vi "daqio_Create_Default_Dashboard.vi"(8 "error in":errorcluster, 11 "daq.io type in":T1={"daq.io ref"=refnum, "daq.io API Base"="http://dashboard.daq.io/api/v1", "Device Key"="", "Account ID"="", "online"=TRUE, "SSL"=TRUE, "buffer"=TRUE}) -> (0 "error out":errorcluster, 2 "Dashboard URL":string, 3 "daq.io type out":T1={"daq.io ref"=refnum, "daq.io API Base"="http://dashboard.daq.io/api/v1", "Device Key"="", "Account ID"="", "online"=TRUE, "SSL"=TRUE, "buffer"=TRUE})   [LabVIEW 2013, in "daqio minimal.lvlib"]
doc: "This VI creates a new default dashboard for a specific account and makes it the new default dashboard for the current device."
uses:
  daqio minimal.lvlib
  _typedefs/daqio-Type.ctl
  <vilib>/httpClient/ClientHandle.ctl
  _typedefs/daqio-Device-Just-Dashboards.ctl
  _typedefs/daqio-Device-Dashboards.ctl
  _typedefs/daqio-Device-Put-Dashboards.ctl
  <vilib>/Easy HTTP Client/Easy HTTP.lvlib
  <vilib>/httpClient/LabVIEWHTTPClient.lvlib
panel:
  out "JSON string":string
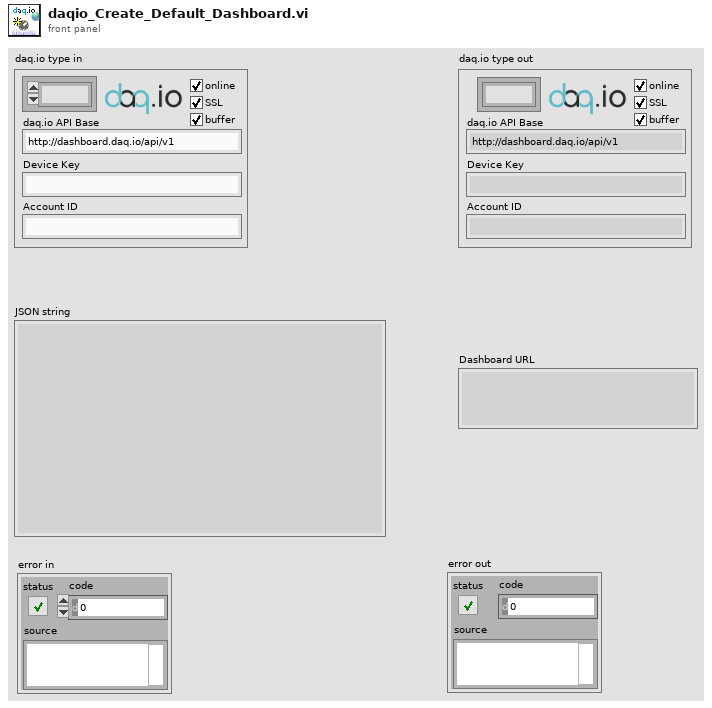
[diagram p1: front panel]
types:
  T1 = typedef "daqio minimal.lvlib/daqio-Type.ctl" = cluster{"daq.io ref":T2, "daq.io API Base":string, "Device Key":string, "Account ID":string, "online":bool, "SSL":bool, "buffer":bool}
  T2 = typedef "LabVIEWHTTPClient.lvlib/ClientHandle.ctl" = refnum<k1>
  T3 = typedef "daqio minimal.lvlib/daqio-Device-Just-Dashboards.ctl" = T4[]
  T4 = typedef "daqio minimal.lvlib/daqio-Device-Dashboards.ctl" = cluster{"active":bool, "definition":string, "_id":string, "label":string}
  T5 = typedef "daqio minimal.lvlib/daqio-Device-Put-Dashboards.ctl" = cluster{"dashboards":T4[]}
  T6 = cluster{"active":bool, "definition":string, "label":string}
  T7 = typedef "daqio minimal.lvlib/daqio-Device-Channels.ctl" = T8[]
  T8 = typedef "daqio minimal.lvlib/daqio-Channels.ctl" = cluster{"key":string, "label":string, "data_type":string, "id":string}
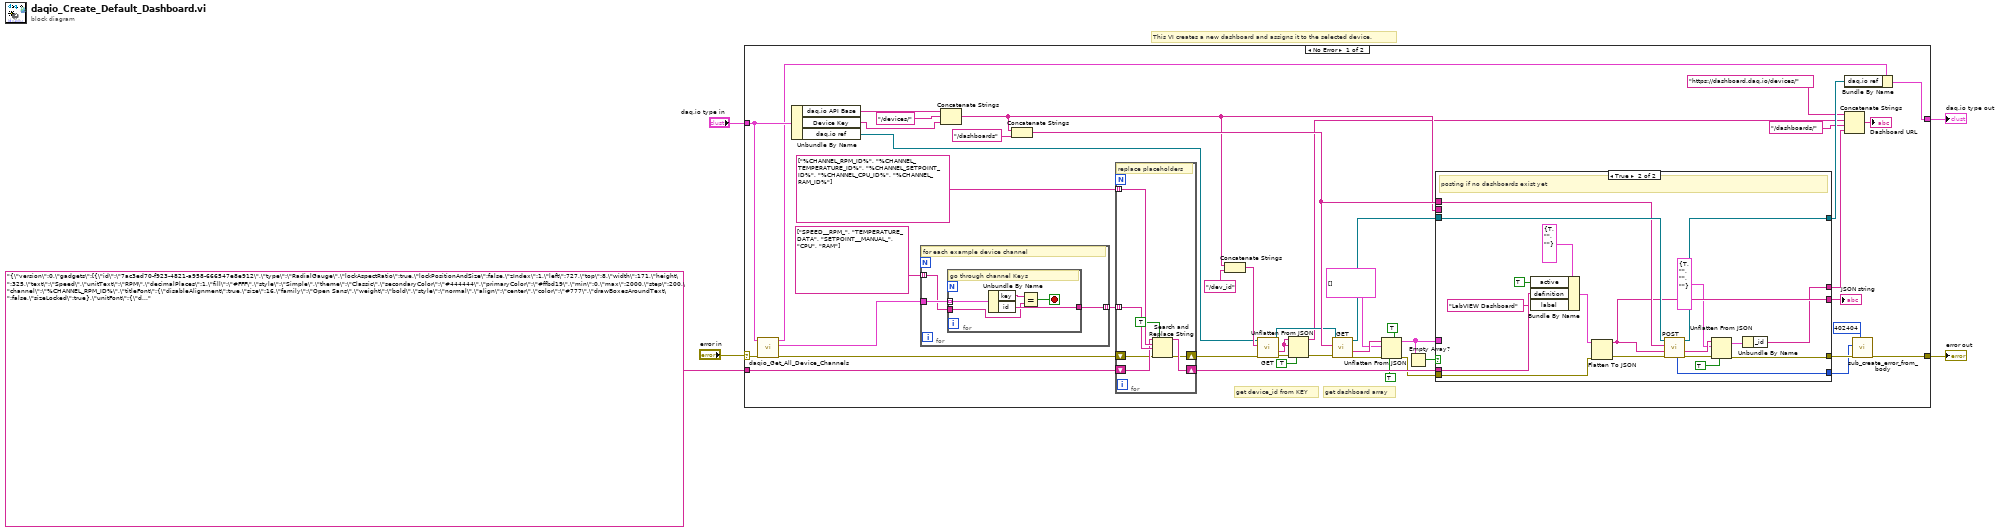
[diagram p0: block diagram]
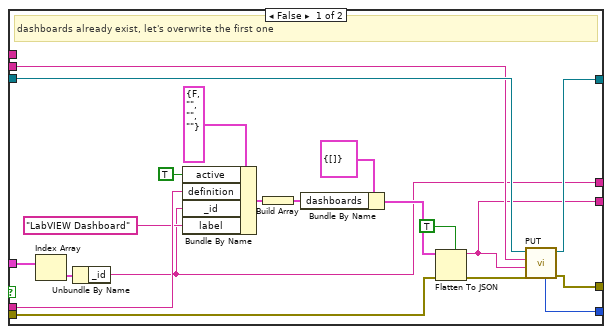
[diagram p2: hidden frame]
diagram:
  # "This VI creates a new dashboard and assigns it to the selected device."
  n1 = case shown="No Error" "error in" {
    selector: "error in" -> [w50 w106]
    tunnel: "daq.io type in" -> [w44 w107]
    tunnel: [w49 w107] -> w4
    tunnel: [w40 w106] -> w3
    tunnel: "{\"version\":0,\"gadgets\":[{\"id\":\"7ac3ed70-f923-4821-a958-666547e8e912\",\"type\":\"RadialGauge\",\"lockAspectRatio\":true,\"lockPositionAndSize\":false,\"zIndex\":1,\"left\":727,\"top\":8,\"width\":171,\"height\":325,\"text\":\"Speed\",\"unitText\":\"RPM\",\"decimalPlaces\":1,\"fill\":\"#FFF\",\"style\":\"Simple\",\"theme\":\"Classic\",\"secondaryColor\":\"#444444\",\"primaryColor\":\"#ffbd19\",\"min\":0,\"max\":2000,\"step\":200,\"channel\":\"%CHANNEL_RPM_ID%\",\"titleFont\":{\"disableAlignment\":true,\"size\":16,\"family\":\"Open Sans\",\"weight\":\"bold\",\"style\":\"normal\",\"align\":\"center\",\"color\":\"#777\",\"drawBoxesAroundText\":false,\"sizeLocked\":true},\"unitFont\":{\"disableAlignment\":true,\"size\":12,\"family\":\"Open Sans\",\"weight\":\"normal\",\"style\":\"normal\",\"align\":\"center\",\"color\":\"#777\",\"drawBoxesAroundText\":true,\"sizeLocked\":true},\"valueFont\":{\"disableAlignment\":true,\"size\":26.71875,\"family\":\"Open Sans\",\"weight\":\"bold\",\"style\":\"normal\",\"align\":\"center\",\"color\":\"#777\",\"drawBoxesAroundText\":false},\"rangeFont\":{\"disableAlignment\":true,\"size\":10.6875,\"family\":\"Open Sans\",\"weight\":\"normal\",\"style\":\"normal\",\"align\":\"center\",\"color\":\"#777\"}},{\"id\":\"7e0172ce-b84d-437a-9326-f0fd3ac7a2ed\",\"type\":\"Image\",\"lockAspectRatio\":true,\"lockPositionAndSize\":false,\"zIndex\":1,\"left\":372,\"top\":231,\"width\":222,\"height\":147,\"image\":\"https://daqio-assets.s3.amazonaws.com/centrifuge_original.png\"},{\"id\":\"4d953908-15d4-4226-91de-77cd2beb7e82\",\"type\":\"Shape\",\"lockAspectRatio\":true,\"lockPositionAndSize\":false,\"zIndex\":0,\"left\":358,\"top\":158,\"width\":254,\"height\":254,\"shape\":\"Circle\",\"strokeWidth\":\"1\",\"stroke\":\"#7a7a7a\",\"fill\":\"#e1e1e1\"},{\"id\":\"c9c26b4d-9cbf-4a0a-b91e-2f65f7344d33\",\"type\":\"Label\",\"lockAspectRatio\":false,\"lockPositionAndSize\":false,\"zIndex\":0,\"left\":346,\"top\":48,\"width\":289,\"height\":70,\"text\":\"Machine Demo\",\"contentFont\":{\"size\":20,\"family\":\"Open Sans\",\"weight\":\"bold\",\"style\":\"normal\",\"align\":\"center\",\"color\":\"#414141\",\"drawBoxesAroundText\":true,\"colorLocked\":true}},{\"id\":\"6d40786f-8469-407d-82b0-a8fb2274aa41\",\"type\":\"Label\",\"lockAspectRatio\":false,\"lockPositionAndSize\":false,\"zIndex\":0,\"left\":374,\"top\":415,\"width\":200,\"height\":67,\"text\":\"Temperature\",\"contentFont\":{\"size\":13,\"family\":\"Open Sans\",\"weight\":\"normal\",\"style\":\"normal\",\"align\":\"center\",\"color\":\"#777\",\"drawBoxesAroundText\":false,\"sizeLocked\":true}},{\"id\":\"cb40a290-c180-4a08-89c5-431a35526d9e\",\"type\":\"HorizontalBar\",\"lockAspectRatio\":true,\"lockPositionAndSize\":false,\"zIndex\":0,\"left\":10,\"top\":111,\"width\":300,\"height\":100,\"text\":\"CPU\",\"unitText\":\"%\",\"decimalPlaces\":1,\"style\":\"Simple\",\"theme\":\"Outline\",\"min\":0,\"max\":100,\"titleFont\":{\"size\":18,\"family\":\"Open Sans\",\"weight\":\"bold\",\"style\":\"normal\",\"align\":\"center\",\"color\":\"#777\",\"drawBoxesAroundText\":false},\"unitFont\":{\"size\":12,\"family\":\"Open Sans\",\"weight\":\"normal\",\"style\":\"normal\",\"align\":\"center\",\"color\":\"#777\",\"drawBoxesAroundText\":true,\"sizeLocked\":true},\"valueFont\":{\"size\":20,\"family\":\"Open Sans\",\"weight\":\"bold\",\"style\":\"normal\",\"align\":\"center\",\"color\":\"#999999\",\"drawBoxesAroundText\":false,\"colorLocked\":true},\"rangeFont\":{\"size\":16,\"family\":\"Open Sans\",\"weight\":\"normal\",\"style\":\"normal\",\"align\":\"center\",\"color\":\"#777\",\"drawBoxesAroundText\":false},\"barColor\":\"#ffd231\",\"channel\":\"%CHANNEL_CPU_ID%\"},{\"id\":\"6f7b8051-d386-4202-81a3-3c12b381a257\",\"type\":\"HorizontalBar\",\"lockAspectRatio\":true,\"lockPositionAndSize\":false,\"zIndex\":0,\"left\":6,\"top\":220,\"width\":300,\"height\":100,\"text\":\"RAM\",\"unitText\":\"%\",\"decimalPlaces\":1,\"style\":\"Simple\",\"theme\":\"Outline\",\"min\":0,\"max\":100,\"titleFont\":{\"size\":18,\"family\":\"Open Sans\",\"weight\":\"bold\",\"style\":\"normal\",\"align\":\"center\",\"color\":\"#777\",\"drawBoxesAroundText\":false},\"unitFont\":{\"size\":12,\"family\":\"Open Sans\",\"weight\":\"normal\",\"style\":\"normal\",\"align\":\"center\",\"color\":\"#777\",\"drawBoxesAroundText\":true,\"sizeLocked\":true},\"valueFont\":{\"size\":20,\"family\":\"Open Sans\",\"weight\":\"bold\",\"style\":\"normal\",\"align\":\"center\",\"color\":\"#979797\",\"drawBoxesAroundText\":false,\"colorLocked\":true},\"rangeFont\":{\"size\":16,\"family\":\"Open Sans\",\"weight\":\"normal\",\"style\":\"normal\",\"align\":\"center\",\"color\":\"#777\",\"drawBoxesAroundText\":false},\"barColor\":\"#ffd231\",\"channel\":\"%CHANNEL_RAM_ID%\"},{\"id\":\"6e31d9f8-654d-4a90-a645-4c0c01ffefb2\",\"type\":\"RadialGauge\",\"lockAspectRatio\":true,\"lockPositionAndSize\":false,\"zIndex\":1,\"left\":729,\"top\":197,\"width\":171,\"height\":325,\"text\":\"Setpoint\",\"unitText\":\"no unit\",\"decimalPlaces\":1,\"fill\":\"#FFF\",\"style\":\"Simple\",\"theme\":\"Classic\",\"secondaryColor\":\"#444444\",\"primaryColor\":\"#ffbd19\",\"min\":0,\"max\":160,\"step\":20,\"channel\":\"%CHANNEL_SETPOINT_ID%\",\"titleFont\":{\"disableAlignment\":true,\"size\":16,\"family\":\"Open Sans\",\"weight\":\"bold\",\"style\":\"normal\",\"align\":\"center\",\"color\":\"#777\",\"drawBoxesAroundText\":false,\"sizeLocked\":true},\"unitFont\":{\"disableAlignment\":true,\"size\":0,\"family\":\"Open Sans\",\"weight\":\"normal\",\"style\":\"normal\",\"align\":\"center\",\"color\":\"#777\",\"drawBoxesAroundText\":false},\"valueFont\":{\"disableAlignment\":true,\"size\":26.71875,\"family\":\"Open Sans\",\"weight\":\"bold\",\"style\":\"normal\",\"align\":\"center\",\"color\":\"#777\",\"drawBoxesAroundText\":false},\"rangeFont\":{\"disableAlignment\":true,\"size\":10.6875,\"family\":\"Open Sans\",\"weight\":\"normal\",\"style\":\"normal\",\"align\":\"center\",\"color\":\"#777\"}},{\"id\":\"90ba8f3d-be02-42b1-90c0-ea490e721fa7\",\"type\":\"Image\",\"lockAspectRatio\":true,\"lockPositionAndSize\":false,\"zIndex\":0,\"left\":441,\"top\":5,\"width\":92,\"height\":61,\"image\":\"https://daqio-assets.s3.amazonaws.com/daq.io_small.png\"},{\"id\":\"03293aae-fb6d-482e-9e2c-42fb101fcfef\",\"type\":\"HorizontalChart\",\"lockAspectRatio\":false,\"lockPositionAndSize\":false,\"zIndex\":0,\"left\":49,\"top\":473,\"width\":853,\"height\":219,\"channels\":[\"%CHANNEL_TEMPERATURE_ID%\"],\"chartType\":\"Line\",\"historyLength\":50,\"enableTimestamps\":false,\"title\":\"Live Data\",\"animation\":false,\"bezierCurve\":false,\"showScale\":true,\"showScaleLabels\":true,\"fillColor\":\"rgba(151,187,205,0.2)\",\"strokeColor\":\"rgba(151,187,205,1)\",\"pointColor\":\"rgba(151,187,205,1)\",\"pointDot\":false,\"datasetFill\":false},{\"id\":\"b5cbcedc-313a-4162-af99-101f51513c83\",\"type\":\"Label\",\"lockAspectRatio\":false,\"lockPositionAndSize\":false,\"zIndex\":0,\"left\":327,\"top\":102,\"width\":319,\"height\":34,\"text\":\"Type: $TYPE\",\"contentFont\":{\"size\":20,\"family\":\"Open Sans\",\"weight\":\"bold\",\"style\":\"normal\",\"align\":\"center\",\"color\":\"#777\",\"drawBoxesAroundText\":false}}],\"background\":\"#FFF\",\"aspectRatio\":\"1280x720\"}" -> [w45 _]
    frame No Error {
      # "get dashboard array"
      # "get device_id from KEY"
      n2 = call "daqio_Get_All_Device_Channels.vi"("error in (no error)"=w50, "daq.io type in"=w44) -> ("error out"=w42:errorcluster, "Device Channels"=w48:T7, "daq.io type out"=w43:T1)  [unwired: 7 in]
      n3 = Unbundle By Name(w44) -> ("daq.io API Base"=w39:string, "Device Key"=w37:string, "daq.io ref"=w16:T2)
      n4 = for {
        tunnel: w48 -> [w100]
        tunnel: string[] ["SPEED__RPM_", "TEMPERATURE_DATA", "SETPOINT__MANUAL_", "CPU", "RAM"] -> [w99] mode=indexing
        tunnel: [w98] -> w22 mode=indexing
        # "for each example device channel"
        n5 = for {
          tunnel: [w105] -> w98
          tunnel: w100 -> [w104] mode=indexing
          tunnel: w99 -> [w103]
          stop <- w101 stop-if-true
          # "go through channel Keys"
          n6 = Unbundle By Name(w104) -> ("key"=w102:string, "id"=w105:string)
          n7 = Equal?(x=w102, y=w103) -> (x = y?=w101:bool)
        }
      }
      n8 = Concatenate Strings(w39, "/devices/" ("string"), w37) -> (w19:string)
      n9 = Concatenate Strings(w19, "/dashboards") -> (w24:string)
      n10 = for {
        tunnel: w22 -> [w97] mode=indexing
        tunnel: string[] ["%CHANNEL_RPM_ID%", "%CHANNEL_TEMPERATURE_ID%", "%CHANNEL_SETPOINT_ID%", "%CHANNEL_CPU_ID%", "%CHANNEL_RAM_ID%"] -> [w96] mode=indexing
        shift-right: [w94] -> w36
        shift-left: w45 -> [w95]
        shift-right: [w92] -> w18
        shift-left: w42 -> [w93]
        # "replace placeholders"
        n11 = Search and Replace String(replace all?=TRUE ("replace all? (F)"), input string=w95, search string=w96, replace string=w97, error in=w93) -> (result string=w94:string, error out=w92:errorcluster)  [unwired: 3 in, 2 out]
      }
      n12 = Concatenate Strings(w19, "/dev_id" ("string")) -> (w17:string)
      n13 = call <vilib>:"GET.vi"("error in (no error)"=w18, "url"=w17, "client handle"=w16) -> ("error out"=w7:errorcluster, "body"=w10:string, "client handle out"=w15:T2)  [unwired: 4 in, 2 out]
      n14 = Unflatten From JSON(JSON string=w10, type and defaults=w10, default null elements? (F)=TRUE, error in (no error)=w7) -> (value=w9:string, error out=w6:errorcluster)  [unwired: 3 in]
      n15 = call <vilib>:"GET.vi"("error in (no error)"=w6, "url"=w24, "client handle"=w15) -> ("error out"=w32:errorcluster, "body"=w35:string, "client handle out"=w30:T2)  [unwired: 4 in, 2 out]
      n16 = Unflatten From JSON(enable LabVIEW extensions? (T)=TRUE, JSON string=w35, type and defaults=T3 [] ("dashboards"), default null elements? (F)=TRUE, error in (no error)=w32) -> (value=w26:T3, error out=w31:errorcluster)  [unwired: 2 in]
      n17 = Empty Array?(array=w26) -> (empty?=w11:bool)
      n18 = case shown="True" w11 {
        tunnel: w36 -> [w68 w90]
        tunnel: w26 -> [w65 _]
        tunnel: w31 -> [w58 w82]
        tunnel: w30 -> [w64 w88]
        tunnel: w19 -> [w63 _]
        tunnel: [w62 w77] -> w29
        tunnel: [w61 w83] -> w28
        tunnel: [w60 w84] -> w27
        tunnel: [w55 w85] -> w25
        tunnel: w24 -> [_ w87]
        tunnel: [w52 w80] -> w12
        frame False {
          # "dashboards already exist, let's overwrite the first one"
          n19 = Index Array(array=w65) -> (element=w66:T4)  [unwired: 1 in]
          n20 = Unbundle By Name(w66) -> ("_id"=w52:string)
          n21 = Bundle By Name(cluster=T4 {"active"=FALSE, "definition"="", "_id"="", "label"=""} ("dashboard"), "active"=TRUE, "definition"=w68, "_id"=w52, "label"="LabVIEW Dashboard") -> (w69:T4)
          n22 = Build Array(w69) -> (w71:T4[])
          n23 = Bundle By Name(cluster=T5 {"dashboards"=[]} ("Device"), "dashboards"=w71) -> (w59:T5)
          n24 = Flatten To JSON(enable LabVIEW extensions? (T)=TRUE, anything=w59, error in (no error)=w58) -> (JSON string=w55:string, 11:w57:errorcluster)
          n25 = call <vilib>:"PUT.vi"("error in (no error)"=w57, "data"=w55, "url"=w63, "client handle"=w64) -> ("error out"=w62:errorcluster, "client handle out"=w60:T2, "HTTP Response Code"=w61:i32)  [unwired: 3 in, 2 out]
        }
        frame True {
          # "posting if no dashboards exist yet"
          n26 = Bundle By Name(cluster=T6 {"active"=TRUE, "definition"="", "label"=""} ("dashboard"), "active"=TRUE, "definition"=w90, "label"="LabVIEW Dashboard") -> (w81:T6)
          n27 = Flatten To JSON(anything=w81, error in (no error)=w82) -> (JSON string=w85:string, 11:w86:errorcluster)  [unwired: 1 in]
          n28 = call <vilib>:"POST.vi"("error in (no error)"=w86, "data"=w85, "url"=w87, "client handle"=w88) -> ("error out"=w78:errorcluster, "body"=w75:string, "client handle out"=w84:T2, "HTTP Response Code"=w83:i32)  [unwired: 3 in, 1 out]
          n29 = Unflatten From JSON(JSON string=w75, type and defaults=T4 {"active"=TRUE, "definition"="", "_id"="", "label"=""} ("dashboard"), default null elements? (F)=TRUE, error in (no error)=w78) -> (value=w76:T4, error out=w77:errorcluster)  [unwired: 3 in]
          n30 = Unbundle By Name(w76) -> ("_id"=w80:string)
        }
      }
      "JSON string" <- w25
      n31 = Bundle By Name(cluster=w43, "daq.io ref"=w27) -> (w49:T1)
      n32 = Concatenate Strings("https://dashboard.daq.io/devices/" ("string"), w9, "/dashboards/" ("string"), w12) -> (→"Dashboard URL":string)
      n33 = call "sub_create_error_from_body.vi"("error code"=402404, "error in (no error)"=w29, "http code"=w28) -> ("error out"=w40:errorcluster)  [unwired: 8 in]
    }
    frame Error {
    }
  }
  "error out" <- w3
  "daq.io type out" <- w4
